vi "carregando.vi"() -> ()   [LabVIEW 2016]
uses:
  numero_imagens.vi
panel:
  out "Calibrando Membros ....":u8(slide) scale=0.0..1700.0
  # "Aguarde"
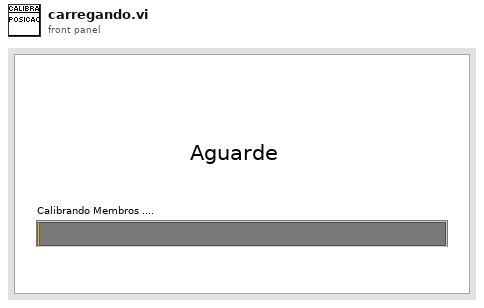
[diagram p1: front panel]
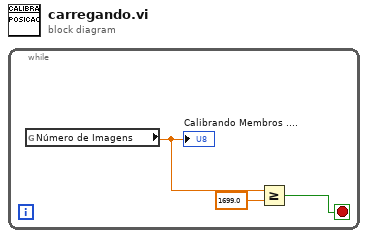
[diagram p0: block diagram]
diagram:
  n1 = while {
    stop <- w1 stop-if-true
    n2 = global read "numero_imagens.vi" "Número de Imagens"() -> (w3:dbl)
    "Calibrando Membros ...." <- w3
    n3 = Greater Or Equal?(x=w3, y=1699.0) -> (x >= y?=w1:bool)
  }
